vi "ble_cmd_gap_connect_direct.vi"(4 "Address Type":T1=1 items=["Public", "Random"], 5 "Connection Interval Max (95ms)":u16=95, 6 "Latency(0)":u16, 7 "Connection Interval Min (75ms)":u16=75, 8 "error in (no error)":errorcluster, 9 "Timeout(1000ms)":u16=1000, 10 "MAC Address":string, 11 "COM Bluegiga in":refnum<visa-resource-name>) -> (0 "error out":errorcluster, 3 "COM Bluegiga out":refnum<visa-resource-name>)   [LabVIEW 2013]
uses:
  type_def/address_type.ctl
  type_def/message_class.ctl
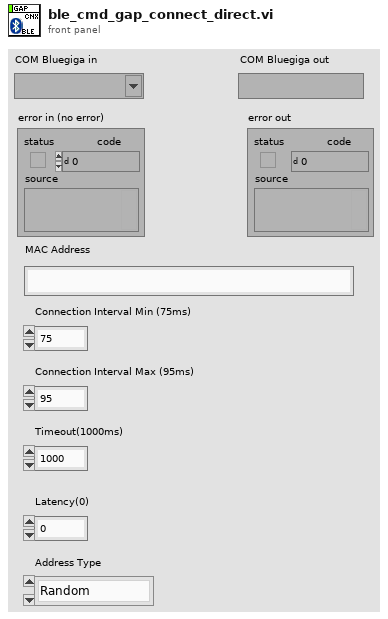
[diagram p1: front panel]
types:
  T1 = typedef "address_type.ctl" = u8
  T2 = typedef "message_class.ctl" = u8
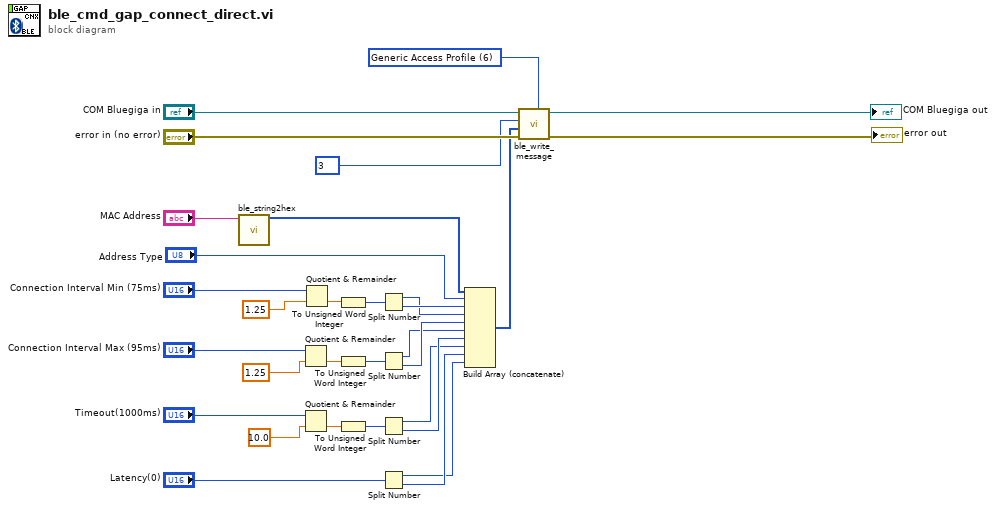
[diagram p0: block diagram]
diagram:
  w7 = T2 6 items=["System", "Persistent Store", "Attribute database", "Connection", "Attribute client", "Security Manager", "Generic Access Profile", "Hardware"] ("Command Class (System)")
  n1 = call "ble_string2hex.vi"("HEX string IN"="MAC Address") -> ("Byte Array IN (index0 LS byte)"=w1:u8[])  [unwired: 10 in]
  n2 = Quotient & Remainder(x="Connection Interval Max (95ms)", y=1.25) -> (floor(x/y)=w24:dbl)  [unwired: 1 out]
  n3 = Quotient & Remainder(x="Timeout(1000ms)", y=10.0) -> (floor(x/y)=w15:dbl)  [unwired: 1 out]
  n4 = Quotient & Remainder(x="Connection Interval Min (75ms)", y=1.25) -> (floor(x/y)=w25:dbl)  [unwired: 1 out]
  n5 = To Unsigned Word Integer(number=w25) -> (unsigned 16bit integer=w23:u16)
  n6 = To Unsigned Word Integer(number=w24) -> (unsigned 16bit integer=w20:u16)
  n7 = To Unsigned Word Integer(number=w15) -> (unsigned 16bit integer=w16:u16)
  n8 = Split Number(x=w23) -> (hi(x)=w21:u8, lo(x)=w22:u8)
  n9 = Split Number(x=w20) -> (hi(x)=w18:u8, lo(x)=w19:u8)
  n10 = Split Number(x=w16) -> (hi(x)=w11:u8, lo(x)=w12:u8)
  n11 = Split Number(x="Latency(0)") -> (hi(x)=w9:u8, lo(x)=w10:u8)
  n12 = Build Array (concatenate)(w1, "Address Type", w22, w21, w19, w18, w12, w11, w10, w9) -> (w17:T1[])
  n13 = call "ble_write_message.vi"("Command Class (System)"=w7, "error in (no error)"="error in (no error)", "Payload(Empty)"=w17, "Message ID (0x00)"=u8 3, "COM Bluegiga in"="COM Bluegiga in") -> ("error out"=→"error out":errorcluster, "COM Bluegiga out"=→"COM Bluegiga out":refnum<visa-resource-name>)  [unwired: 4 in, 1 out]
